vi "Update Value.vi"(6 "Time":dbl, 8 "error in (no error)":errorcluster, 11 "SystemConfigStatusIndicator in":refnum<class "SystemConfigStatusIndicator.lvclass">) -> (0 "error out":errorcluster, 1 "Update":bool, 2 "Value":variant, 3 "SystemConfigStatusIndicator out":refnum<class "SystemConfigStatusIndicator.lvclass">)   [LabVIEW 2020, in "VolatusGUIElements.lvlib" / "SystemConfigStatusIndicator.lvclass"]
uses:
  SystemConfigStatusIndicator.lvclass
  Volatus/ConfigMonitorInfoValue/ConfigMonitorInfoValue.lvclass
  C:/dev/lv20CE/relink/lv-promises/Promises/Value/Value.lvclass
  SystemConfigStatusIndicator.lvclass/SystemConfigStatusIndicator.ctl
  Volatus/MessageQ/MessageQ.lvclass
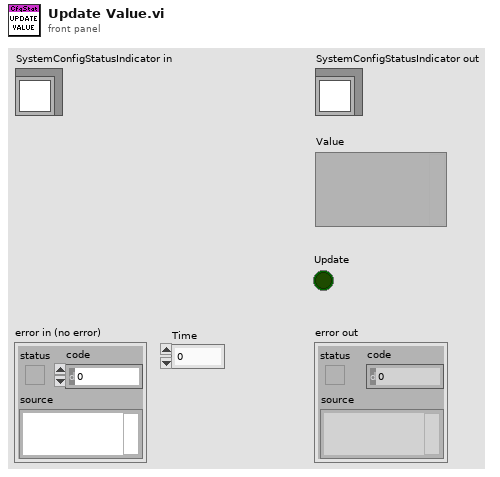
[diagram p1: front panel]
types:
  T1 = typedef "Volatus.lvlib/Config Monitor Module.lvclass/Node Config Info.ctl" = cluster{"Node":string, "Config Version":string, "Config Hash":string, "Pull":bool, "Push":bool, "Version Color":u32, "Hash Color":u32, "Node Color":u32}
  T2 = cluster{"Status Color":u32, "Status String":string, "Config GUI":bool, "Status":cluster{"Node Name":string, "Node Color":u32, "Version Color":u32, "Hash Color":u32}[]}
  T3 = cluster{"Node Name":string, "Node Color":u32, "Version Color":u32, "Hash Color":u32}
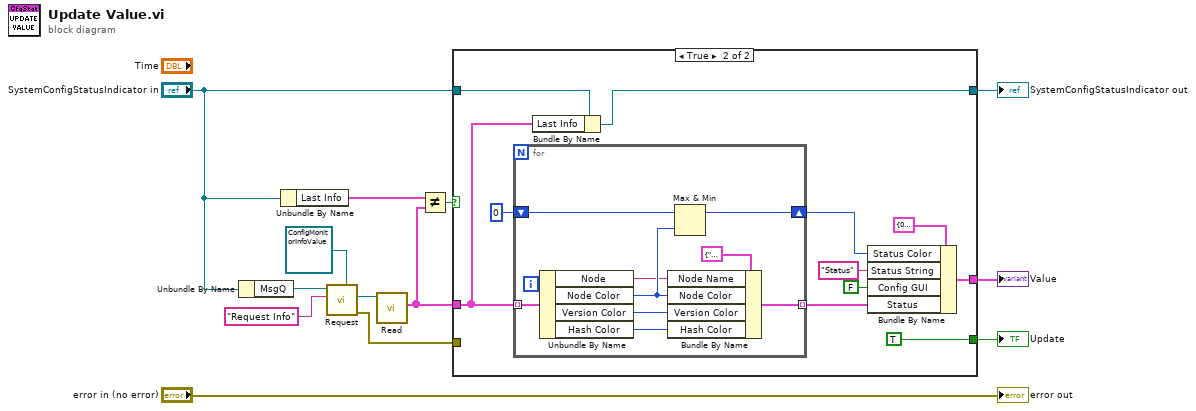
[diagram p0: block diagram]
diagram:
  n1 = Unbundle By Name("SystemConfigStatusIndicator in") -> ("MsgQ"=w12:refnum<class "MessageQ.lvclass">)
  n2 = Unbundle By Name("SystemConfigStatusIndicator in") -> ("Last Info"=w6:T1[])
  n3 = call "Request.vi"("Response Value Type"=refnum<class "ConfigMonitorInfoValue.lvclass"> refnum ("Volatus:ConfigMonitorInfoValue.lvclass"), "ID"="Request Info", "MessageQ in"=w12) -> ("error out"=w1:errorcluster, "Response"=w9:refnum<class "ConfigMonitorInfoValue.lvclass">)  [unwired: 6 in, 1 out]
  n4 = call "Read.vi"("ConfigMonitorInfoValue in"=w9) -> ("Info"=w7:T1[])  [unwired: 10 in]
  n5 = Not Equal?(x=w6, y=w7) -> (x != y?=w4:bool)
  n6 = case shown="True" w4 {
    tunnel: [_ w20] -> w8
    tunnel: w7 -> [_ w17]
    tunnel: "SystemConfigStatusIndicator in" -> [w14 w18]
    tunnel: [w14 w16] -> w3
    tunnel: [_ TRUE] -> w2
    tunnel: w1 -> [_ _]
    frame False {
    }
    frame True {
      n7 = for {
        tunnel: [w33] -> w23 mode=indexing
        tunnel: w17 -> [w32] mode=indexing
        shift-right: [w27] -> w21
        shift-left: u32 0 -> [w28]
        n8 = Unbundle By Name(w32) -> ("Node"=w26:string, "Node Color"=w29:u32, "Version Color"=w31:u32, "Hash Color"=w30:u32)
        n9 = Bundle By Name(cluster=T3 {"Node Name"="", "Node Color"=0, "Version Color"=0, "Hash Color"=0} ("Node Status"), "Node Name"=w26, "Node Color"=w29, "Version Color"=w31, "Hash Color"=w30) -> (w33:T3)
        n10 = Max & Min(x=w28, y=w29) -> (max(x,y)=w27:u32)  [unwired: 1 out]
      }
      n11 = Bundle By Name(cluster=w18, "Last Info"=w17) -> (w16:refnum<class "SystemConfigStatusIndicator.lvclass">)
      n12 = Bundle By Name(cluster=T2 {"Status Color"=0, "Status String"="", "Config GUI"=FALSE, "Status"=[]} ("System Config Status"), "Status Color"=w21, "Status String"="Status", "Config GUI"=FALSE, "Status"=w23) -> (w20:T2)
    }
  }
  "SystemConfigStatusIndicator out" <- w3
  "Value" <- w8
  "Update" <- w2
  "error out" <- "error in (no error)"
